vi "A-K separation.vi"(4 "Input wave":waveform(dbl)) -> (0 "Katod wave (inverted)":waveform(dbl), 1 "Anod wave":waveform(dbl))   [LabVIEW 2012]
uses:
  <vilib>/measure/NI_MABase.lvlib
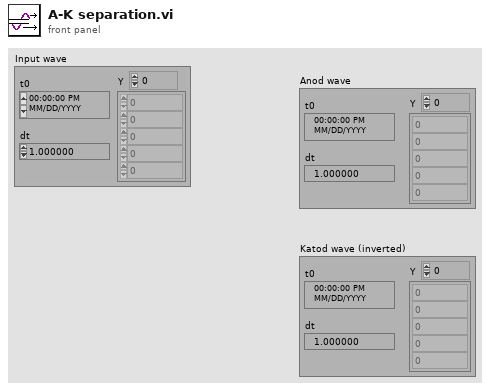
[diagram p1: front panel]
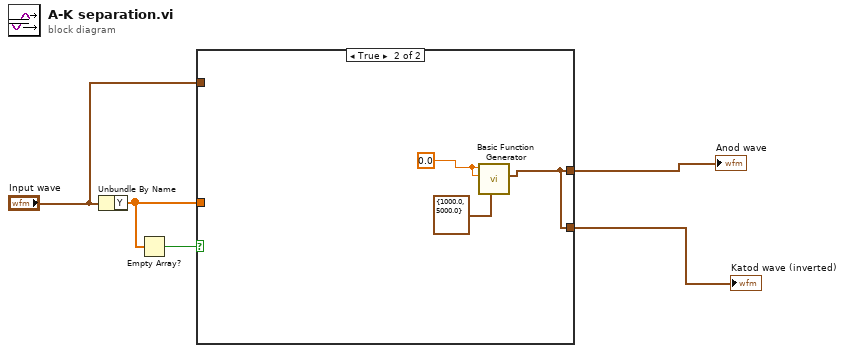
[diagram p0: block diagram]
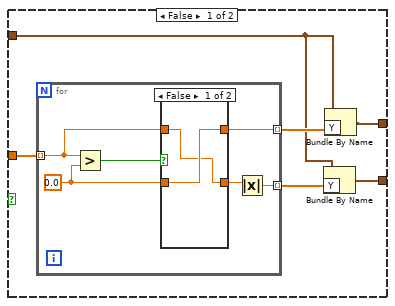
[diagram p2: hidden frame]
diagram:
  n1 = Unbundle By Name("Input wave") -> ("Y"=w5:dbl[])
  n2 = Empty Array?(array=w5) -> (empty?=w4:bool)
  n3 = case shown="True" w4 {
    tunnel: w5 -> [w11 _]
    tunnel: [w10 w22] -> w3
    tunnel: [w9 w22] -> w2
    tunnel: "Input wave" -> [w6 _]
    frame False {
      n4 = for {
        tunnel: w11 -> [w16] mode=indexing
        tunnel: [w15] -> w7 mode=indexing
        tunnel: [w12] -> w8 mode=indexing
        w14 = 0.0 ("y")
        n5 = Greater?(x=w16, y=w14) -> (0:w17:bool)
        n6 = case shown="False" w17 {
          tunnel: w16 -> [w18 w21]
          tunnel: [w19 w21] -> w15
          tunnel: [w18 w20] -> w13
          tunnel: w14 -> [w19 w20]
          frame False {
          }
          frame True {
          }
        }
        n7 = Absolute Value(x=w13) -> (abs(x)=w12:dbl)
      }
      n8 = Bundle By Name(cluster=w6, "Y"=w8) -> (w9:waveform(dbl))
      n9 = Bundle By Name(cluster=w6, "Y"=w7) -> (w10:waveform(dbl))
    }
    frame True {
      w24 = 0.0 ("frequency")
      n10 = call <vilib>:"Basic Function Generator.vi"("sampling info"=cluster{"Fs":dbl, "#s":dbl} {"Fs"=1000.0, "#s"=5000.0}, "amplitude"=w24, "frequency"=w24) -> ("signal out"=w22:waveform(dbl))  [unwired: 6 in, 2 out]
    }
  }
  "Anod wave" <- w3
  "Katod wave (inverted)" <- w2
